vi "Open.vi"(8 "error in (no error)":errorcluster, 11 "VISA resource name":refnum<visa-resource-name>) -> (0 "error out":errorcluster, 3 "VISA resource":refnum<visa-resource-name>)   [LabVIEW 2019, in "KH7008.lvlib"]
uses:
  KH7008.lvlib
  <vilib>/Instr/_visa.llb/VISA Configure Serial Port (Instr).vi
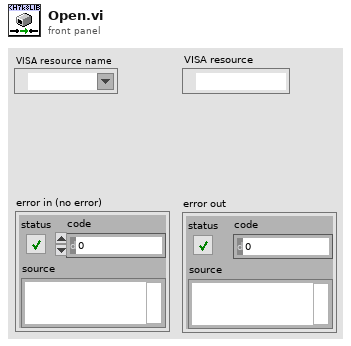
[diagram p1: front panel]
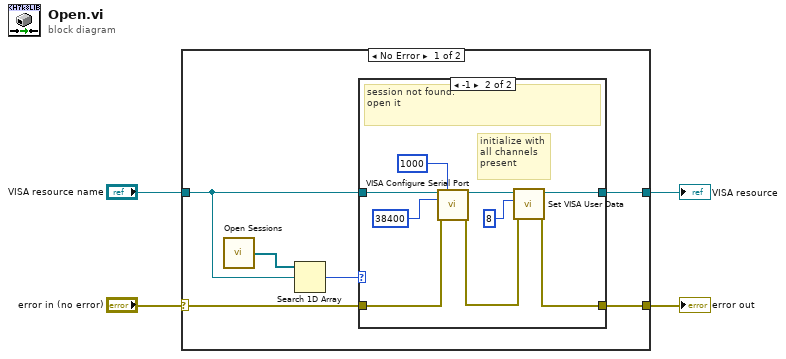
[diagram p0: block diagram]
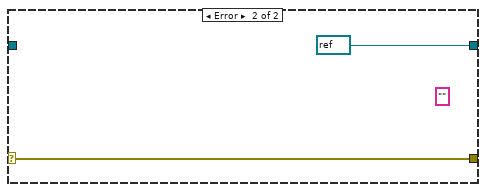
[diagram p3: hidden frame]
diagram:
  n1 = case shown="No Error" "error in (no error)" {
    selector: "error in (no error)" -> [w9 w23]
    tunnel: [w6 refnum<visa-resource-name> refnum ("VISA resource name out")] -> w4
    tunnel: [w5 w23] -> w3
    tunnel: "VISA resource name" -> [w8 _]
    frame No Error {
      n2 = call <vilib>:"Open Sessions.vi"() -> ("Array of Refnums"=w10:refnum<visa-resource-name>[])  [unwired: 2 in]
      n3 = Search 1D Array(1D array=w10, element=w8) -> (index of element=w7:i32)  [unwired: 1 in]
      n4 = case shown="-1" w7 {
        tunnel: [w12 w17] -> w6
        tunnel: [w11 w16] -> w5
        tunnel: w9 -> [w11 w20]
        tunnel: w8 -> [w12 w19]
        frame 0, Default {
          # "session found:\ndo not open again"
        }
        frame -1 {
          # "initialize with\nall channels\npresent"
          # "session not found:\nopen it"
          n5 = call-poly "VISA Configure Serial Port"("VISA resource name"=w19, "timeout (10sec)"=u32 1000, "baud rate (9600)"=u32 38400, "error in (no error)"=w20) -> ("VISA resource name out"=w18:refnum<visa-resource-name>, "error out"=w15:errorcluster)  [unwired: 5 in, 5 out]
          n6 = call "Set VISA User Data.vi"("error in (no error)"=w15, "User Data"=8, "VISA Refnum in"=w18) -> ("error out"=w16:errorcluster, "VISA Refnum out"=w17:refnum<visa-resource-name>)  [unwired: 7 in]
        }
      }
    }
    frame Error {
      (unwired) "" ("SR")
    }
  }
  "VISA resource" <- w4
  "error out" <- w3
